vi "Tab Setup.vi"(8 "error in (no error)":errorcluster, 9 "EXTERNAL MICROCONTROLLER":refnum<visa-resource-name>, 10 "GRBL COM PORT":refnum<visa-resource-name>, 11 "TabControl in":refnum<vi>) -> (0 "error out":errorcluster, 3 "Cluster":T1)   [LabVIEW 2021]
uses:
  <vilib>/Instr/_visa.llb/VISA Configure Serial Port (Instr).vi
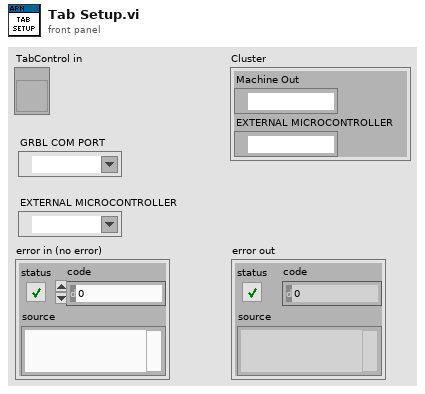
[diagram p1: front panel]
types:
  T1 = cluster{"Machine Out":refnum<visa-resource-name>, "EXTERNAL MICROCONTROLLER":refnum<visa-resource-name>}
  T2 = enum32{"Serial Configuration", "GCODE", "Manual Overide", "Tune"}
  T3 = cluster{"VISA resource name out":refnum<visa-resource-name>, "EXTERNAL MICROCONTROLLER":refnum<visa-resource-name>}
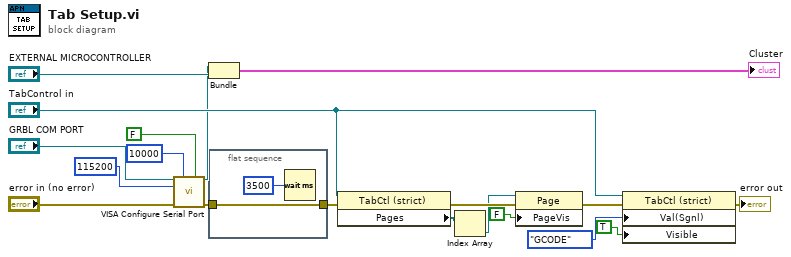
[diagram p0: block diagram]
diagram:
  n1 = call-poly "VISA Configure Serial Port"("VISA resource name"="GRBL COM PORT", "timeout (10sec)"=u32 10000, "Enable Termination\nChar (T)"=FALSE ("Enable Termination\nChar (T)"), "baud rate (9600)"=u32 115200, "error in (no error)"="error in (no error)") -> ("VISA resource name out"=w5:refnum<visa-resource-name>, "error out"=w3:errorcluster)  [unwired: 9 in]
  n2 = Bundle("VISA resource name out"=w5, "EXTERNAL MICROCONTROLLER"="EXTERNAL MICROCONTROLLER") -> (→"Cluster":T3)  [unwired: 1 in]
  n3 = flat-sequence {
    tunnel: w3 -> [w21]
    tunnel: [w21] -> w2
    frame #0 {
      n4 = Wait (ms)(milliseconds to wait=u32 3500) -> ()  [unwired: 1 out]
    }
  }
  n5 = property on="Property Node" class="TabCtl (strict)"(reference="TabControl in", error in=w2) -> (error out=w16:errorcluster, "Pages"=w13:refnum<vi>[])  [unwired: 1 out]
  n6 = Index Array(array=w13) -> (element=w14:refnum<vi>)  [unwired: 1 in]
  n7 = property class="Page"(reference=w14, error in=w16, "PageVis"=FALSE ("Page Visible")) -> (error out=w17:errorcluster)  [unwired: 1 out]
  n8 = property on="Property Node" class="TabCtl (strict)"(reference="TabControl in", error in=w17, "Val(Sgnl)"=T2."GCODE" ("Value (Signaling)"), "Visible"=TRUE) -> (error out=→"error out":errorcluster)  [unwired: 1 out]
